vi "Open Module Main Front Panel.vi"(7 "App Instance":refnum<vi>, 8 "error in":errorcluster, 11 "Library in":refnum<class "Library.lvclass">) -> (0 "error out":errorcluster, 3 "Library out":refnum<class "Library.lvclass">)   [LabVIEW 2020, in "Panther Dashboard.lvlib" / "Library.lvclass"]
uses:
  Library.lvclass
  C:/GitClones/PantherDashboard/src/LabVIEW/Panther Dashboard/Class/LabVIEWItem/LabVIEWItem.lvclass
  LabVIEWItem/LabVIEWItem.lvclass/LabVIEWItem.ctl
  LabVIEWItem/Read Item Path.vi
  Library.lvclass/Library.ctl
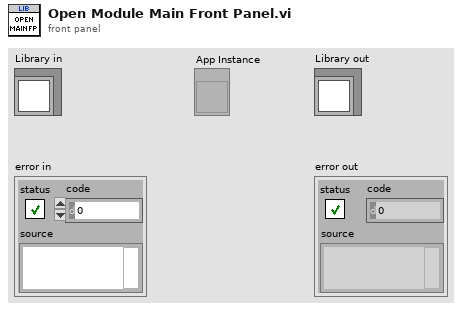
[diagram p1: front panel]
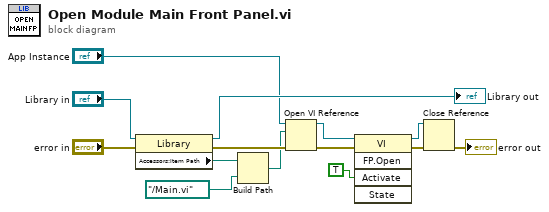
[diagram p0: block diagram]
diagram:
  n1 = property class="Library"(reference="Library in", error in="error in") -> (reference out=→"Library out":refnum<class "Library.lvclass">, error out=w11:errorcluster, "Accessors:Item Path"=w9:path)
  n2 = Build Path(base path=w9, name or relative path=path "../Main.vi") -> (appended path=w3:path)
  n3 = Open VI Reference(application reference (local)="App Instance", vi path=w3, error in (no error)=w11) -> (vi reference=w5:refnum<vi>, error out=w12:errorcluster)  [unwired: 3 in]
  n4 = invoke class="VI" method="FP.Open"(reference=w5, error in=w12, "Activate"=TRUE ("Activate?")) -> (reference out=w4:refnum<vi>, error out=w13:errorcluster)  [unwired: 2 in, 3 out]
  n5 = Close Reference(reference=w4, error in (no error)=w13) -> (error out=→"error out":errorcluster)
